vi "公式写入.vi"(5 "临界滴定数":dbl format="%#_13g", 7 "公式":cluster{"X^2":dbl, "X":dbl, "b":dbl}, 8 "error in (no error)":errorcluster caption="错误输入（无错误）", 9 "量程":enum16{"低量程1", "低量程2", "高量程1", "高量程2"}(ring), 10 "测量模式":T1(ring), 11 "测量参数":enum16{"CODMn"}(ring)) -> (0 "error out":errorcluster caption="错误输出")   [LabVIEW 2016]
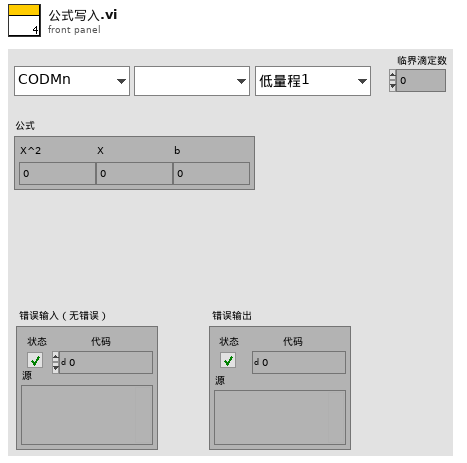
[diagram p1: front panel]
types:
  T1 = enum16{"", "水样测量", "标样核查", "零点核查", "跨度核查", "空白测试", "平行样测试", "加标回收"}
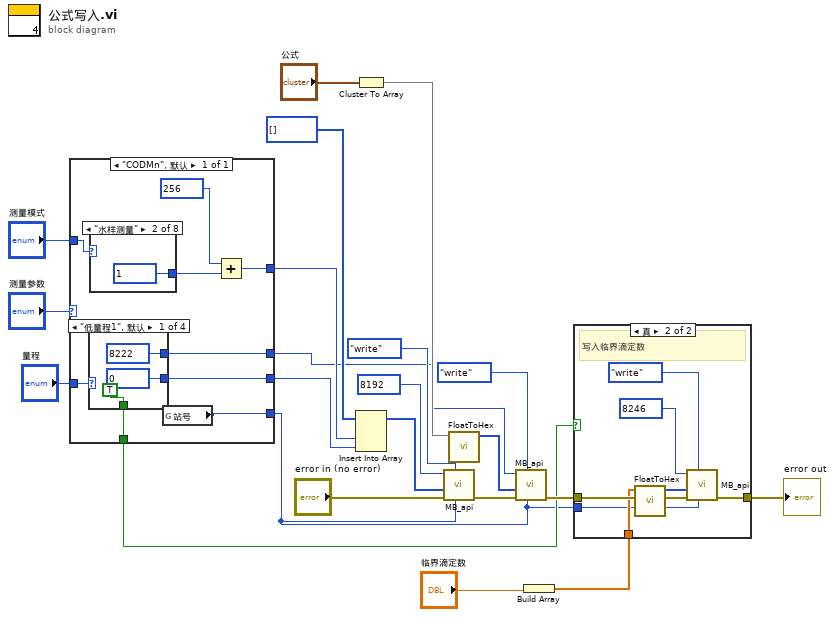
[diagram p0: block diagram]
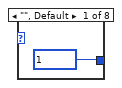
[diagram p3: hidden frame]
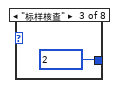
[diagram p4: hidden frame]
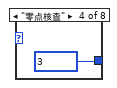
[diagram p5: hidden frame]
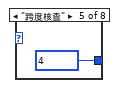
[diagram p6: hidden frame]
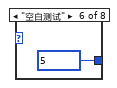
[diagram p7: hidden frame]
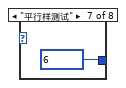
[diagram p8: hidden frame]
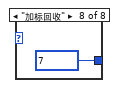
[diagram p9: hidden frame]
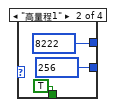
[diagram p10: hidden frame]
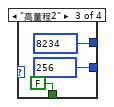
[diagram p11: hidden frame]
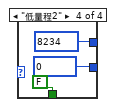
[diagram p12: hidden frame]
diagram:
  n1 = case shown="\"CODMn\", 默认" "测量参数" {
    tunnel: "测量模式" -> [w26]
    tunnel: "量程" -> [w31]
    tunnel: [w27] -> w1
    tunnel: [w28] -> w16
    tunnel: [w30] -> w15
    tunnel: [w24] -> w5
    tunnel: [w23] -> w4
    frame "CODMn", Default {
      n2 = case shown="\"低量程1\", 默认" w31 {
        tunnel: [u16 0 ("starting address") u16 256 ("starting address") u16 256 ("starting address") u16 0 ("starting address")] -> w30
        tunnel: [u16 8222 ("starting address") u16 8222 ("starting address") u16 8234 ("starting address") u16 8234 ("starting address")] -> w24
        tunnel: [TRUE TRUE FALSE FALSE] -> w23
        frame "低量程1", Default {
        }
        frame "高量程1" {
        }
        frame "高量程2" {
        }
        frame "低量程2" {
        }
      }
      n3 = case shown="\"水样测量\"" w26 {
        tunnel: [u16 1 ("starting address") u16 1 ("starting address") u16 2 ("starting address") u16 3 ("starting address") u16 4 ("starting address") u16 5 ("starting address") u16 6 ("starting address") u16 7 ("starting address")] -> w25
        frame "", Default {
        }
        frame "水样测量" {
        }
        frame "标样核查" {
        }
        frame "零点核查" {
        }
        frame "跨度核查" {
        }
        frame "空白测试" {
        }
        frame "平行样测试" {
        }
        frame "加标回收" {
        }
      }
      n4 = global read "挥发酚断电保存全局变量.vi" "站号"() -> (w27:u16)
      n5 = Add(x=u16 256 ("starting address"), y=w25) -> (x+y=w28:u16)
    }
  }
  n6 = Cluster To Array(cluster="公式") -> (array=w21:dbl[])
  n7 = Insert Into Array(array=u16[] [] ("数组"), new element #1=w16, new element #2=w15) -> (w9:u16[])  [unwired: 1 in]
  n8 = call "MB_api.vi"("Slave ID"=w1, "STEP"=enum16{"open", "read", "write", "close"}."write", "Error in"="error in (no error)", "values"=w9, "starting address"=u16 8192) -> ("error out"=w12:errorcluster)  [unwired: 4 in, 2 out]
  n9 = call "FloatToHex.vi"("浮点数"=w21) -> ("DCBA整形输出"=w8:u16[])  [unwired: 10 in]
  n10 = call "MB_api.vi"("Slave ID"=w1, "STEP"=enum16{"open", "read", "write", "close"}."write", "Error in"=w12, "values"=w8, "starting address"=w5) -> ("error out"=w7:errorcluster)  [unwired: 4 in, 2 out]
  n11 = Build Array("临界滴定数") -> (w3:dbl[])
  n12 = case shown="真" w4 {
    tunnel: w7 -> [w52 w57]
    tunnel: [w52 w56] -> w6
    tunnel: w3 -> [_ w54]
    tunnel: w1 -> [_ w53]
    frame False {
    }
    frame True {
      # "写入临界滴定数"
      n13 = call "FloatToHex.vi"("浮点数"=w54) -> ("DCBA整形输出"=w55:u16[])  [unwired: 10 in]
      n14 = call "MB_api.vi"("Slave ID"=w53, "STEP"=enum16{"open", "read", "write", "close"}."write", "Error in"=w57, "values"=w55, "starting address"=u16 8246) -> ("error out"=w56:errorcluster)  [unwired: 4 in, 2 out]
    }
  }
  "error out" <- w6
